vi "rs3 configure all.vi"(0 "Select Resolution":u16, 5 "Sensor in":u64, 7 "Stream selection":u16(ring) items=["Depth + Left Color", "Unrectified L + R", "Rectified L + R", "Depth Only", "RGB ext. Only", "Depth + L Monochrome"], 11 "error in (no error)":errorcluster) -> (1 "Output stream L":T1, 2 "Sensor out":u64, 3 "number of modes":u16, 4 "config error":string, 8 "Output stream":string[](array[string]), 10 "extrin out":T2={"rotation[0]"=1.0, "rotation[1]"=0.0, "rotation[2]"=0.0, "rotation[3]"=0.0, "rotation[4]"=1.0, "rotation[5]"=0.0, "rotation[6]"=0.0, "rotation[7]"=0.0, "rotation[8]"=1.0, "translation[0]"=-0.053904004, "translation[1]"=0.0, "translation[2]"=0.0}, 12 "Output Stream R":T1, 13 "L-R Baseline, mm":sgl, 14 "Stream Profile Handles":u64[](array[numeric]), 15 "error out":errorcluster)   [LabVIEW 2017, in "libRealSense3.lvlib"]
doc: "This VI configures the CAMERA-SENSOR to stream a specific set of 2 PROFILES.\n\nSteam selection: \nDepth+Left Color, \nUnrectified Left + Right (The raw input images)\nRectified Left + Right\n\nThe output array of STREAM PROFILE HANDLES is used to START the streams.\n\nThis VI also returns the BASELINE of the stereo module."
uses:
  libRealSense3.lvlib
panel:
  out "Profiles_list_out":u64
  out "Profiles count":i32
  out "Stream Profile Array":T3(array[cluster]) {"model" items=["RS_DISTORTION_NONE", "RS_DISTORTION_MODIFIED_BROWN_CONRADY", "RS_DISTORTION_INVERSE_BROWN_CONRADY", "RS_DISTORTION_FTHETA", "RS_DISTORTION_BROWN_CONRADY", "RS_DISTORTION_COUNT"]; "RS Stream" items=["    RS2_STREAM_ANY,", "    RS2_STREAM_DEPTH                            , /**< Native stream of depth data produced by RealSense device */", "    RS2_STREAM_COLOR                            , /**< Native stream of color data captured by RealSense device */", "    RS2_STREAM_INFRARED                         , /**< Native stream of infrared data captured by RealSense device */", "    RS2_STREAM_FISHEYE                          , /**< Native stream of fish-eye (wide) data captured from the dedicate motion camera */", "    RS2_STREAM_GYRO                             , /**< Native stream of gyroscope motion data produced by RealSense device */", "    RS2_STREAM_ACCEL                            , /**< Native stream of accelerometer motion data produced by RealSense device */", "    RS2_STREAM_GPIO                             , /**< Signals from external device connected through GPIO */", "    RS2_STREAM_COUNT"]; "RS Format" items=["    RS2_FORMAT_ANY             , /**< When passed to enable stream, librealsense will try to provide best suited format */", "    RS2_FORMAT_Z16             , /**< 16-bit linear depth values. The depth is meters is equal to depth scale * pixel value. */", "    RS2_FORMAT_DISPARITY16     , /**< 16-bit linear disparity values. The depth in meters is equal to depth scale / pixel value. */", "    RS2_FORMAT_XYZ32F          , /**< 32-bit floating point 3D coordinates. */", "    RS2_FORMAT_YUYV            , /**< Standard YUV pixel format as described in https://en.wikipedia.org/wiki/YUV */", "    RS2_FORMAT_RGB8            , /**< 8-bit red, green and blue channels */", "    RS2_FORMAT_BGR8            , /**< 8-bit blue, green, and red channels -- suitable for OpenCV */", "    RS2_FORMAT_RGBA8           , /**< 8-bit red, green and blue channels + constant alpha channel equal to FF */", "    RS2_FORMAT_BGRA8           , /**< 8-bit blue, green, and red channels + constant alpha channel equal to FF */", "    RS2_FORMAT_Y8              , /**< 8-bit per-pixel grayscale image */", "    RS2_FORMAT_Y16             , /**< 16-bit per-pixel grayscale image */", "    RS2_FORMAT_RAW10           , /**< Four 10-bit luminance values encoded into a 5-byte macropixel */", "    RS2_FORMAT_RAW16           , /**< 16-bit raw image */", "    RS2_FORMAT_RAW8            , /**< 8-bit raw image */", "    RS2_FORMAT_UYVY            , /**< Similar to the standard YUYV pixel format, but packed in a different order */", "    RS2_FORMAT_MOTION_RAW      , /**< Raw data from the motion sensor */", "    RS2_FORMAT_MOTION_XYZ32F   , /**< Motion data packed as 3 32-bit float values, for X, Y, and Z axis */", "    RS2_FORMAT_GPIO_RAW        , /**< Raw data from the external sensors hooked to one of the GPIO's */", "    RS2_FORMAT_COUNT             /**< Number of enumeration values. Not a valid input: intended to be used in for-loops. */"]}
  # "RS3 Configure All"
  # "(C) Intel Corp.,  AGJ 2017"
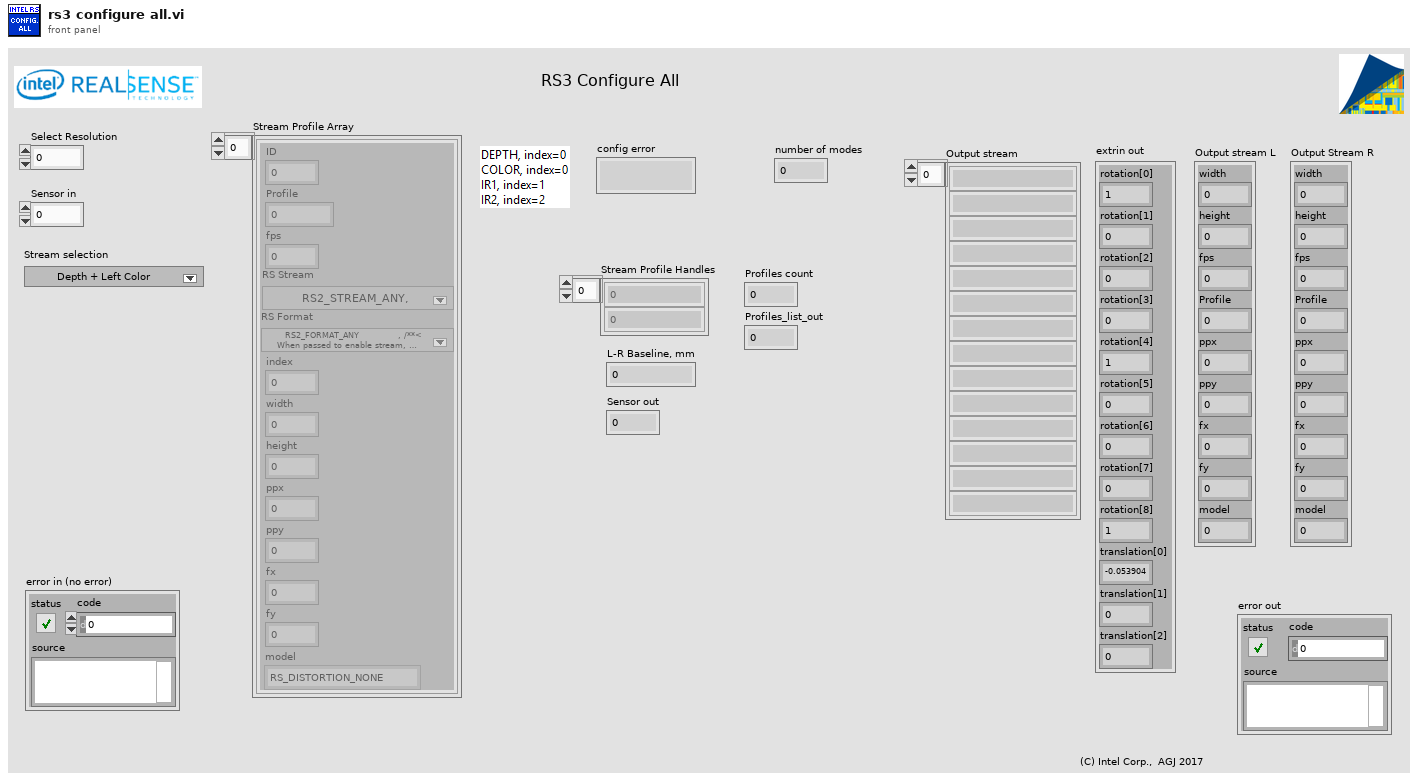
[diagram p1: front panel]
types:
  T1 = cluster{"width":i32, "height":i32, "fps":i32, "Profile":u64, "ppx":sgl, "ppy":sgl, "fx":sgl, "fy":sgl, "model":u32}
  T2 = cluster{"rotation[0]":sgl, "rotation[1]":sgl, "rotation[2]":sgl, "rotation[3]":sgl, "rotation[4]":sgl, "rotation[5]":sgl, "rotation[6]":sgl, "rotation[7]":sgl, "rotation[8]":sgl, "translation[0]":sgl, "translation[1]":sgl, "translation[2]":sgl}
  T3 = cluster{"ID":i32, "Profile":u64, "fps":i32, "RS Stream":u16, "RS Format":u16, "index":u16, "width":u16, "height":u16, "ppx":sgl, "ppy":sgl, "fx":sgl, "fy":sgl, "model":u32}[]
  T4 = cluster{"ID":i32, "Profile":u64, "fps":i32, "RS Stream":u16, "RS Format":u16, "index":u16, "width":u16, "height":u16, "ppx":sgl, "ppy":sgl, "fx":sgl, "fy":sgl, "model":u32}
  T5 = cluster{"width":i32, "height":i32, "ppx":sgl, "ppy":sgl, "fx":sgl, "fy":sgl, "model":u32, "coeffs[0]":sgl, "coeffs[1]":sgl, "coeffs[2]":sgl, "coeffs[3]":sgl, "coeffs[4]":sgl}
  T6 = cluster{"width":i32, "height":i32, "fps":i32, "Profile":u64, "ppx":sgl, "ppy":sgl, "fx":sgl, "fy":sgl, "model":u32}[]
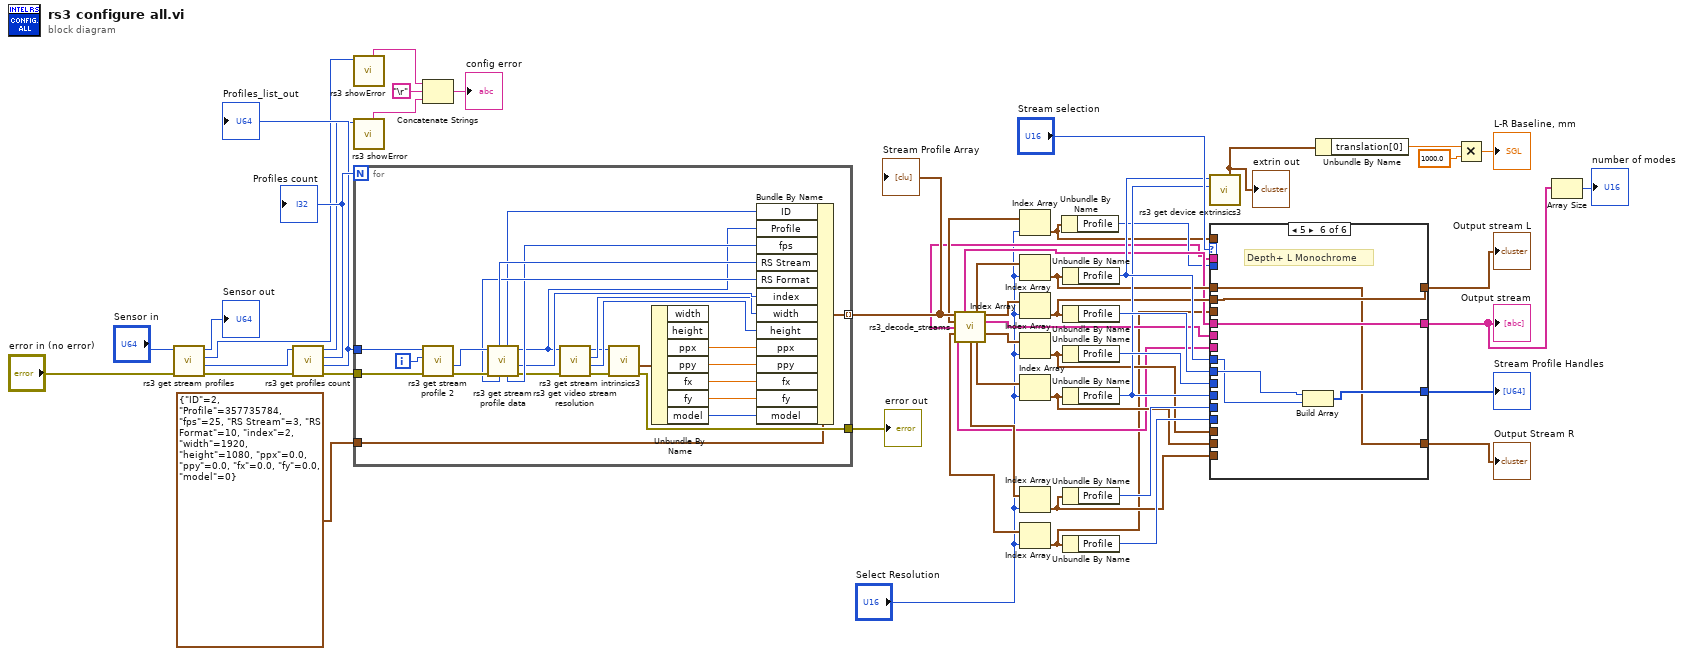
[diagram p0: block diagram]
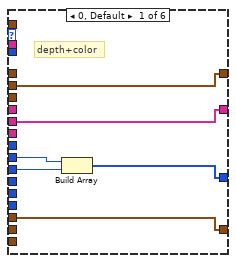
[diagram p2: hidden frame]
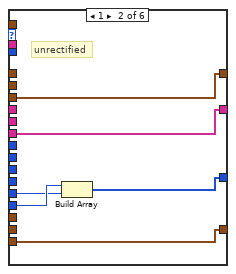
[diagram p3: hidden frame]
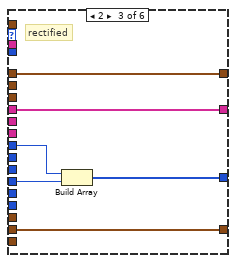
[diagram p4: hidden frame]
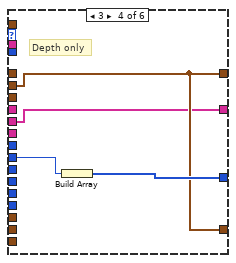
[diagram p5: hidden frame]
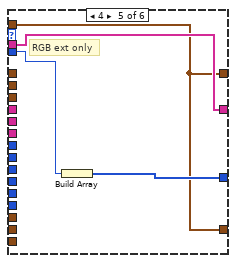
[diagram p6: hidden frame]
diagram:
  n1 = call "rs3 get stream profiles.vi"("error in (no error)"="error in (no error)", "Sensor in"="Sensor in") -> (0:"error out"=w42:errorcluster, "Stream profile list"=w41:u64, 2:"error out"=w40:u64, "Sensor out"=→"Sensor out":u64)  [unwired: 6 in]
  n2 = call "rs3 get profiles count.vi"("error in"=w42, "Profiles_list"=w41) -> ("error out"=w44:errorcluster, "Profiles_list_out"=w45:u64, "Profiles count"=w46:i32, "error"=w43:u64)  [unwired: 6 in]
  "Profiles count" <- w46
  "Profiles_list_out" <- w45
  n3 = call "rs3 showError.vi"("error"=w40) -> ("Error summary"=w38:string)  [unwired: 6 in, 4 out]
  n4 = call "rs3 showError.vi"("error"=w43) -> ("Error summary"=w36:string)  [unwired: 6 in, 4 out]
  n5 = for {
    N: w46 -> [_]
    tunnel: w44 -> [w78]
    tunnel: w45 -> [w77]
    tunnel: T4 {"ID"=2, "Profile"=357735784, "fps"=25, "RS Stream"=3, "RS Format"=10, "index"=2, "width"=1920, "height"=1080, "ppx"=0.0, "ppy"=0.0, "fx"=0.0, "fy"=0.0, "model"=0} ("output cluster") -> [w59]
    tunnel: [w68] -> w33 mode=indexing
    tunnel: [w61] -> w51
    i -> [w76]
    n6 = call "rs3 get stream profile 2.vi"("error in (no error)"=w78, "index"=w76, "Stream Profile list in"=w77) -> ("error out"=w74:errorcluster, "stream profile"=w75:u64)  [unwired: 5 in, 2 out]
    n7 = call "rs3 get stream profile data.vi"("error in (no error)"=w74, "Profile"=w75) -> ("error out"=w67:errorcluster, "index"=w69:i32, "Profile out"=w66:u64, "frame rate"=w71:i32, "unique id"=w70:i32, "RS Format"=w72:u16, "RS Stream"=w73:u16)  [unwired: 2 in, 1 out]
    n8 = call "rs3 get video stream resolution.vi"("error in (no error)"=w67, "Profile"=w66) -> ("error out"=w62:errorcluster, "height"=w65:u32, "width"=w64:u32, "Profile out"=w63:u64)  [unwired: 5 in, 1 out]
    n9 = call "rs3 get stream intrinsics3.vi"("error in (no error)"=w62, "stream profile"=w63) -> ("error out"=w61:errorcluster, "intrin out"=w60:T5)  [unwired: 6 in, 2 out]
    n10 = Unbundle By Name(w60) -> ("ppx"=w58:sgl, "ppy"=w57:sgl, "fx"=w56:sgl, "fy"=w55:sgl, "model"=w54:u32)  [unwired: 2 out]
    n11 = Bundle By Name(cluster=w59, "ID"=w70, "Profile"=w66, "fps"=w71, "RS Stream"=w73, "RS Format"=w72, "index"=w69, "width"=w64, "height"=w65, "ppx"=w58, "ppy"=w57, "fx"=w56, "fy"=w55, "model"=w54) -> (w68:T4)
  }
  "error out" <- w51
  "Stream Profile Array" <- w33
  n12 = Concatenate Strings(w38, "\r", w36) -> (→"config error":string)
  n13 = call "rs3_decode_streams.vi"("Stream profile array"=w33) -> ("IR Left Array"=w9:string[], "IR left"=w32:T6, "Depth Stream"=w47:T6, 5:"RGB ext."=w5:T6, "Depth Stream strings"=w11:string[], 7:"RGB ext."=w2:string[], 9:"Unrectified L IR"=w22:T6, "Color Left"=w48:T6, 11:"Unrectified L IR"=w10:string[], "Unrectified R  IR"=w21:T6, "IR Right"=w31:T6)  [unwired: 1 in, 3 out]
  n14 = Index Array(array=w5, index="Select Resolution") -> (element=w3:T1)
  n15 = Index Array(array=w32, index="Select Resolution") -> (element=w13:T1)
  n16 = Index Array(array=w47, index="Select Resolution") -> (element=w18:T1)
  n17 = Index Array(array=w48, index="Select Resolution") -> (element=w17:T1)
  n18 = Index Array(array=w31, index="Select Resolution") -> (element=w14:T1)
  n19 = Index Array(array=w21, index="Select Resolution") -> (element=w12:T1)
  n20 = Index Array(array=w22, index="Select Resolution") -> (element=w8:T1)
  n21 = Unbundle By Name(w3) -> ("Profile"=w4:u64)
  n22 = Unbundle By Name(w13) -> ("Profile"=w24:u64)
  n23 = Unbundle By Name(w18) -> ("Profile"=w49:u64)
  n24 = Unbundle By Name(w17) -> ("Profile"=w50:u64)
  n25 = Unbundle By Name(w14) -> ("Profile"=w23:u64)
  n26 = Unbundle By Name(w12) -> ("Profile"=w19:u64)
  n27 = Unbundle By Name(w8) -> ("Profile"=w20:u64)
  n28 = call "rs3 get device extrinsics3.vi"("Target Stream Profile"=w23, "Origin Stream Profile"=w24) -> ("extrin out"=w30:T2)  [unwired: 7 in, 2 out]
  "extrin out" <- w30
  n29 = case shown="5" "Stream selection" {
    tunnel: [w84 w88 w94 w100 w104 w107] -> w52
    tunnel: w50 -> [w83 _ _ _ _ _]
    tunnel: w49 -> [w82 _ _ w99 _ w109]
    tunnel: w24 -> [_ _ w96 _ _ w108]
    tunnel: w23 -> [_ _ w95 _ _ _]
    tunnel: w20 -> [_ w90 _ _ _ _]
    tunnel: w19 -> [_ w89 _ _ _ _]
    tunnel: w18 -> [w81 _ _ w98 _ w106]
    tunnel: w17 -> [w80 _ _ _ _ _]
    tunnel: [w81 w87 w93 w98 w101 w106] -> w16
    tunnel: [w80 w86 w92 w98 w101 w105] -> w15
    tunnel: w14 -> [_ _ w92 _ _ _]
    tunnel: w13 -> [_ _ w93 _ _ w105]
    tunnel: w12 -> [_ w86 _ _ _ _]
    tunnel: w8 -> [_ w87 _ _ _ _]
    tunnel: w11 -> [w79 _ _ w97 _ _]
    tunnel: [w79 w85 w91 w97 w102 w110] -> w7
    tunnel: w10 -> [_ w85 _ _ _ _]
    tunnel: w9 -> [_ _ w91 _ _ w110]
    tunnel: w4 -> [_ _ _ _ w103 _]
    tunnel: w3 -> [_ _ _ _ w101 _]
    tunnel: w2 -> [_ _ _ _ w102 _]
    frame 0, Default {
      # "depth+color"
      n30 = Build Array(w82, w83) -> (w84:u64[])
    }
    frame 1 {
      # "unrectified"
      n31 = Build Array(w90, w89) -> (w88:u64[])
    }
    frame 2 {
      # "rectified"
      n32 = Build Array(w96, w95) -> (w94:u64[])
    }
    frame 3 {
      # "Depth only"
      n33 = Build Array(w99) -> (w100:u64[])
    }
    frame 4 {
      # "RGB ext only"
      n34 = Build Array(w103) -> (w104:u64[])
    }
    frame 5 {
      # "Depth+ L Monochrome"
      n35 = Build Array(w109, w108) -> (w107:u64[])
    }
  }
  "Stream Profile Handles" <- w52
  "Output stream L" <- w16
  "Output Stream R" <- w15
  "Output stream" <- w7
  n36 = Unbundle By Name(w30) -> ("translation[0]"=w29:sgl)
  n37 = Multiply(x=w29, y=sgl 1000.0) -> (x*y=→"L-R Baseline, mm":sgl)
  n38 = Array Size(array=w7) -> (size(s)=→"number of modes":i32)
